vi "pf_Get_Camera_Property_String.vi"(8 "error in (no error)":errorcluster, 10 "Property Name":string, 11 "IMAQ Session in":refnum<k11>) -> (0 "error out":errorcluster, 1 "String Value":string, 2 "Property Name out":string, 3 "IMAQ Session out":refnum<k11>)   [LabVIEW 2025, in "Photonfocus_Toolkit.lvlib"]
doc: "Gets the value of a String type property."
uses:
  Photonfocus_Toolkit.lvlib
  _Private/Controls/pf_Camera_ctrl_mngr_action.ctl
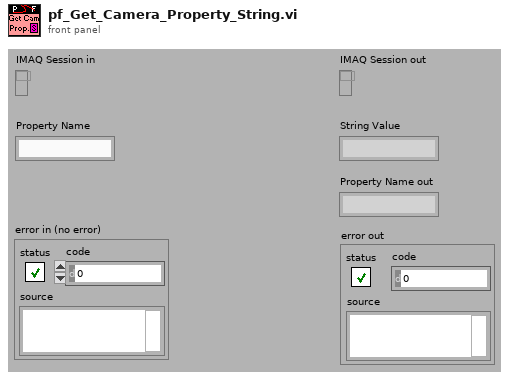
[diagram p1: front panel]
types:
  T1 = typedef "Photonfocus_Toolkit.lvlib/pf_Camera_ctrl_mngr_action.ctl" = enum16{"Create", "Destroy", "Set", "Get"}
  T2 = typedef "Photonfocus_Toolkit.lvlib/pf_Camera_Control.ctl" = cluster{"Port Name":string, "Port Number":i32, "IMAQ Session":refnum<k11>, "PeakDetector_Mode":T3, "Window.W":u32, "Window.H":u32}
  T3 = typedef "Photonfocus_Toolkit.lvlib/pf_PeakDetector_Mode.ctl" = enum16{"Undefined", "2D only", "2D and 3D", "3D only"}
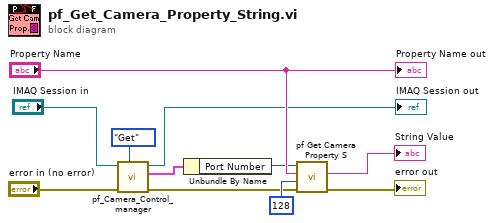
[diagram p0: block diagram]
diagram:
  n1 = call "pf_Camera_Control_manager.vi"("Action"=pf_Camera_ctrl_mngr_action."Get", "error in (no error)"="error in (no error)", "IMAQ Session in"="IMAQ Session in") -> ("error out"=w6:errorcluster, "Camera Control out"=w2:T2, "IMAQ Session out"=→"IMAQ Session out":refnum<k11>)  [unwired: 1 in, 5 out]
  n2 = Unbundle By Name(w2) -> ("Port Number"=w1:i32)
  n3 = call "pf Get Camera Property S.vi"("error in (no error)"=w6, "iSize"=128, "pProperty"="Property Name", "iPort"=w1) -> ("error out"=→"error out":errorcluster, "pValue out"=→"String Value":string)  [unwired: 6 out]
  "Property Name out" <- "Property Name"
